vi "Teleop.vi"(10 "Match Info":T1={"Autonomous Elapsed Seconds"=0.0, "TeleOp Elapsed Seconds"=0.0, "Disabled Elapsed Seconds"=0.0, "Visited Autonomous"=FALSE, "Visited TeleOp"=FALSE, "Visited Disabled"=FALSE, "Autonomous Settings"={"Autonomous Style"=enum."Independent", "VI Refnum"=refnum}}, 11 "Call Context":T2) -> ()   [LabVIEW 2018]
doc: "This VI is called for each TeleOp packet received from the DS where the robot is not disabled. It is often used to read from the joysticks and update I/O or to update setpoints for timed control loops. It should complete and return within 20 milliseconds or it may miss DS packets."
uses:
  <vilib>/Rock Robotics/WPI/DriverStation/WPI_DriverStationDerivedRobotMode.ctl
  <vilib>/Rock Robotics/WPI/DriverStation/WPI_DriverStationMatch Info.ctl
  <vilib>/Rock Robotics/WPI/Utilities/WPI_GetSetVariantRefNum.vi
  <vilib>/Rock Robotics/Network Tables/SD Read Number.vi
panel:
  out "ENCODER VALUE LIFT 2":dbl=20.0 format="%#_13g"
  out "ENCODER VALUE Retractor":dbl=20.0 format="%#_13g"
  out "ENCODER VALUE cLIMBER":dbl=20.0 format="%#_13g"
  out "ENCODER VALUE LIFT":dbl=20.0 format="%#_13g"
  out "BR Current":dbl
  out "FL Current":dbl
  out "BL Current":dbl
  out "lim":bool
  out "Tote Offset":dbl
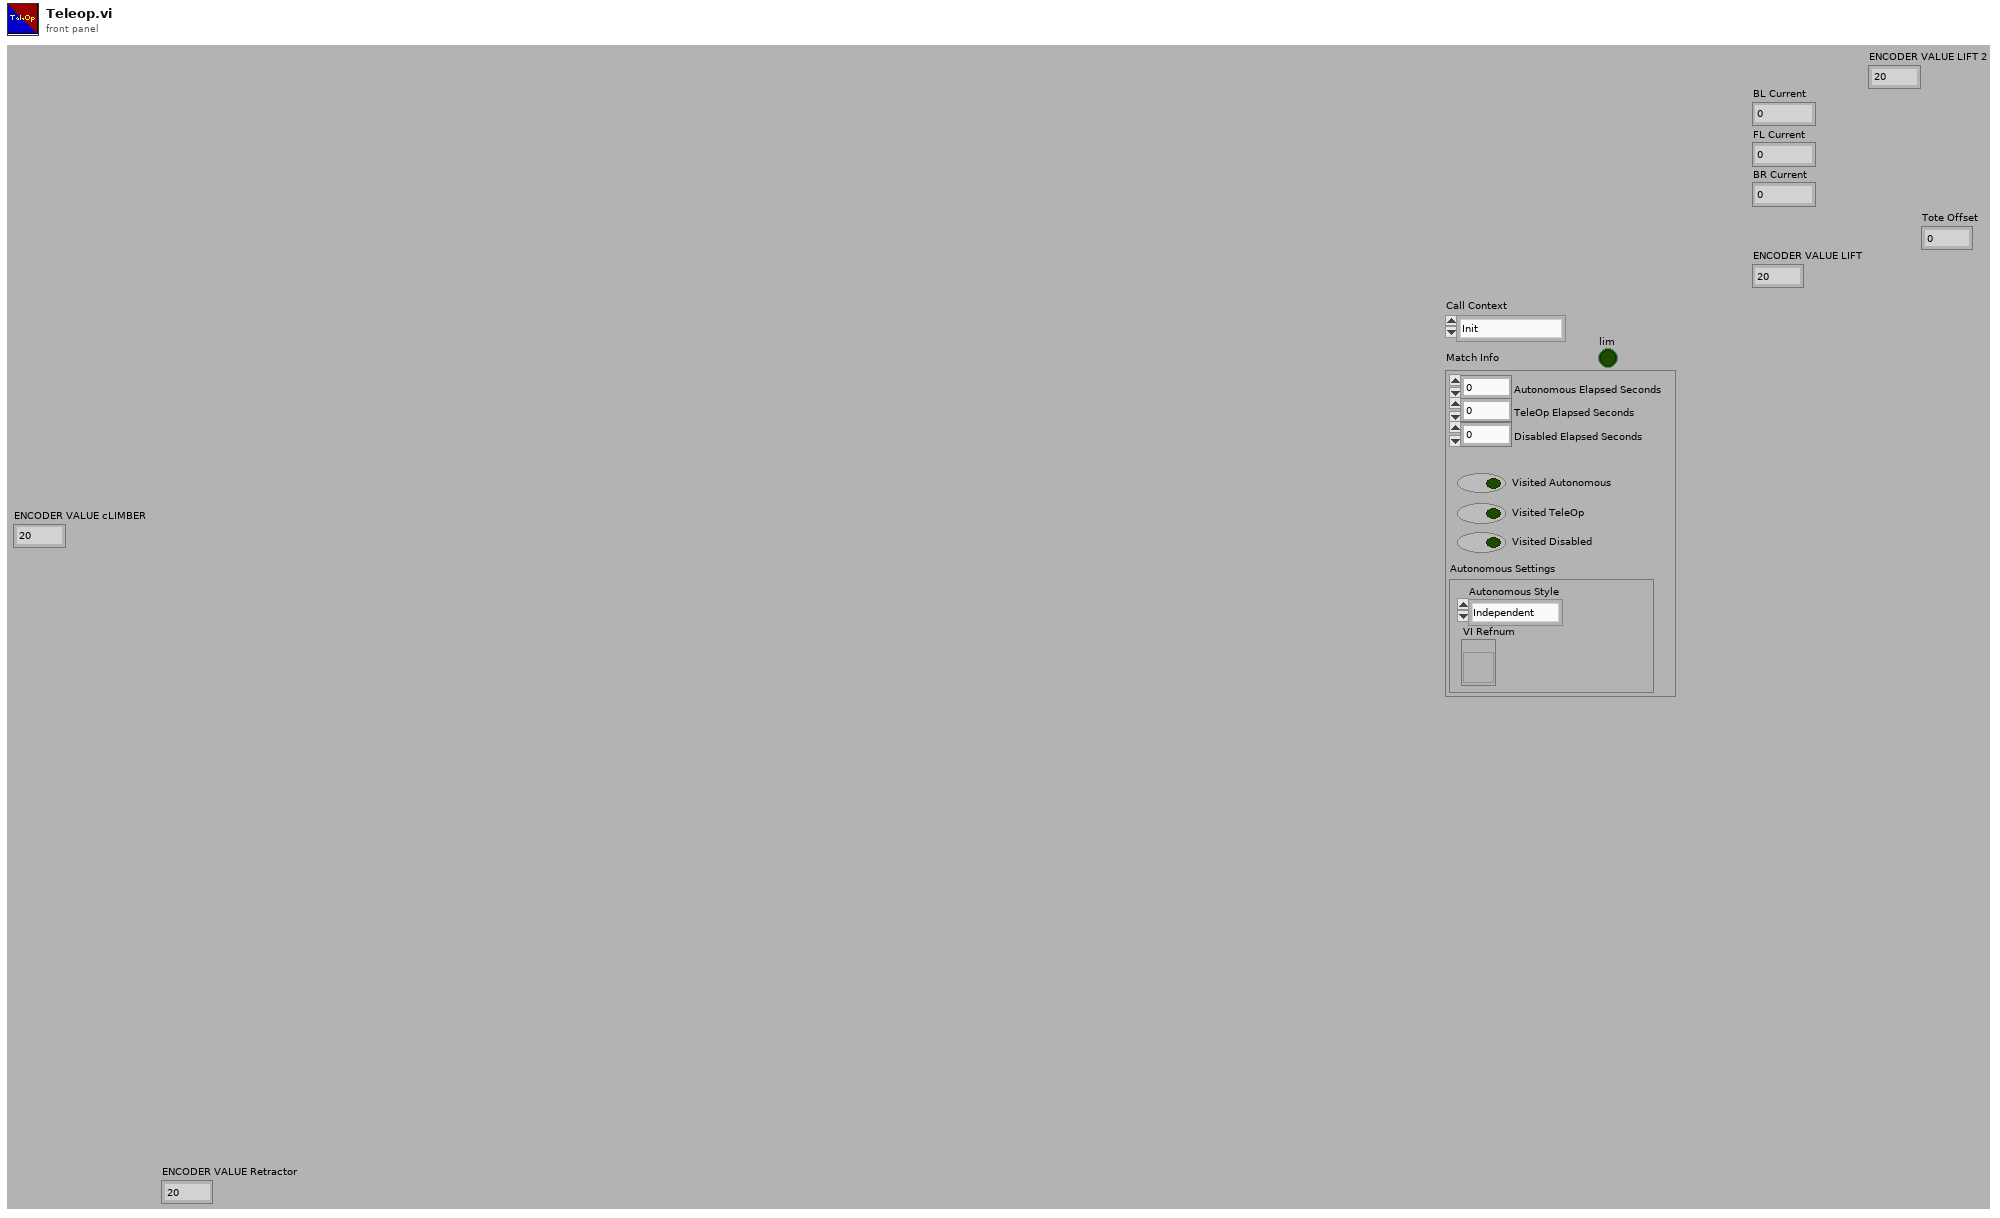
[diagram p1: front panel]
types:
  T1 = typedef "WPI_DriverStationMatch Info.ctl" = cluster{"Autonomous Elapsed Seconds":dbl, "TeleOp Elapsed Seconds":dbl, "Disabled Elapsed Seconds":dbl, "Visited Autonomous":bool, "Visited TeleOp":bool, "Visited Disabled":bool, "Autonomous Settings":cluster{"Autonomous Style":enum16{"Iterative", "Independent"}, "VI Refnum":refnum<vi>}}
  T2 = typedef "WPI_DriverStationDerivedRobotMode.ctl" = enum16{"Init", "Execute", "Stop"}
  T3 = typedef "WPI_JoystickDevRef.ctl" = cluster{"Device":T4}
  T4 = typedef "WPI_JoystickDeviceEnum.ctl" = enum16{"USB 0", "USB 1", "USB 2", "USB 3", "USB 4", "USB 5"}
  T5 = cluster{"Buttons[0]":bool, "Buttons[1]":bool, "Buttons[2]":bool, "Buttons[3]":bool, "Buttons[4]":bool, "Buttons[5]":bool, "Buttons[6]":bool, "Buttons[7]":bool, "Buttons[8]":bool, "Buttons[9]":bool, "Buttons[10]":bool, "Buttons[11]":bool}
  T6 = typedef "WPI_EncoderDevRef.ctl" = cluster{"DevStatus":errorcluster, "EncoderIndex":T7, "CounterIndex":T8, "DistancePerCount":dbl, "Decoding Type":T9}
  T7 = typedef "FPGA_EncoderIdx.ctl" = enum8{"Enc 0", "Enc 1", "Enc 2", "Enc 3", "Enc 4", "Enc 5", "Enc 6", "Enc 7", "Invalid"}
  T8 = typedef "FPGA_CounterCtrSystemIndex.ctl" = enum8{"Ctr 0", "Ctr 1", "Ctr 2", "Ctr 3", "Ctr 4", "Ctr 5", "Ctr 6", "Ctr 7", "Invalid"}
  T9 = typedef "WPI_EncoderType.ctl" = enum16{"1x", "2x", "4x"}
  T10 = cluster{"Buttons[0]":bool, "Buttons[1]":bool, "Buttons[2]":bool, "Buttons[3]":bool, "Buttons[4]":bool, "Buttons[5]":bool, "Buttons[6]":bool, "Buttons[7]":bool, "Buttons[8]":bool, "Buttons[9]":bool}
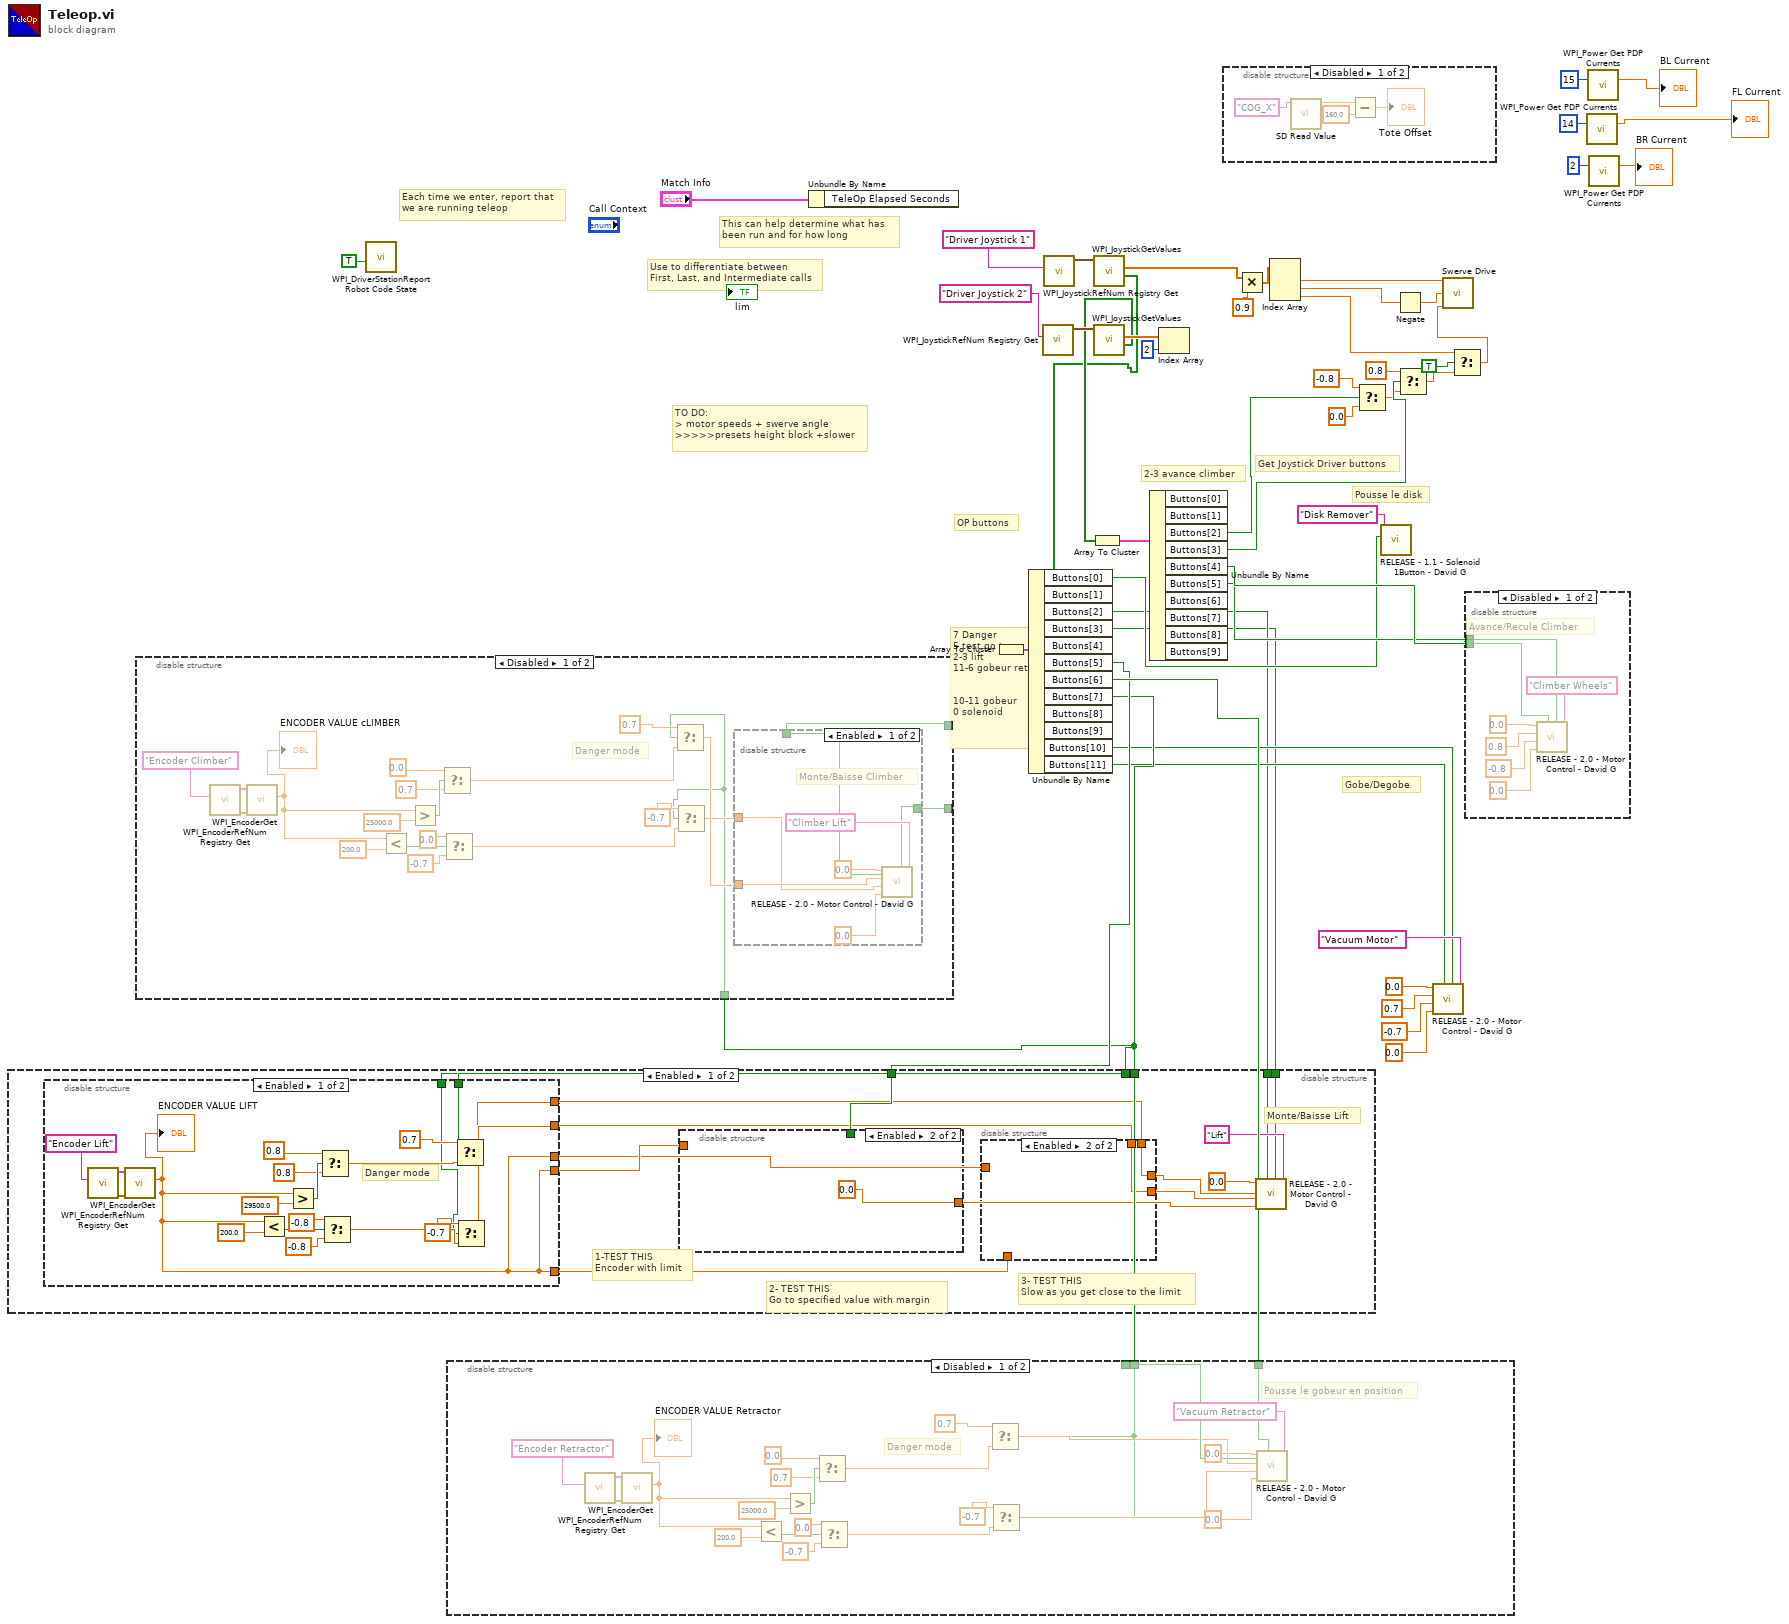
[diagram p0: block diagram]
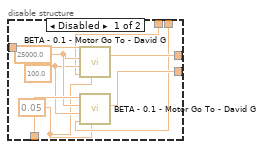
[diagram p7: hidden frame]
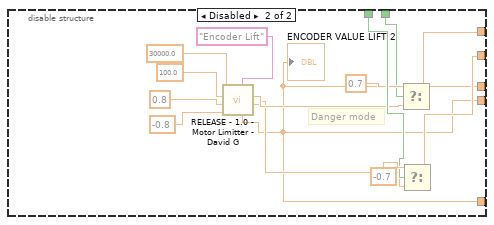
[diagram p8: hidden frame]
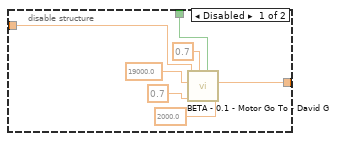
[diagram p9: hidden frame]
diagram:
  # "2-3 avance climber"
  # "7 Danger\n5 test go to\n2-3 lift\n11-6 gobeur retractor\n\n\n10-11 gobeur\n0 solenoid"
  # "OP buttons"
  # "TO DO: \n> motor speeds + swerve angle\n>>>>>presets height block +slower"
  # "Gobe/Degobe"
  # "Pousse le disk"
  # "Get Joystick Driver buttons"
  # "Each time we enter, report that\nwe are running teleop"
  # "Use to differentiate between\nFirst, Last, and Intermediate calls"
  # "This can help determine what has\nbeen run and for how long"
  n1 = call <vilib>:"WPI_DriverStationReport Robot Code State.vi"("TeleOp"=TRUE ("Autonomous")) -> ()  [unwired: 10 in, 1 out]
  n2 = Unbundle By Name("Match Info") -> ()  [unwired: 1 out]
  n3 = call <vilib>:"WPI_JoystickRefNum Registry Get.vi"("refnum name"="Driver Joystick 2") -> ("JoystickDevRef"=w46:T3)  [unwired: 1 in, 9 out]
  n4 = call <vilib>:"WPI_JoystickRefNum Registry Get.vi"("refnum name"="Driver Joystick 1") -> ("JoystickDevRef"=w48:T3)  [unwired: 1 in, 9 out]
  n5 = call <vilib>:"WPI_JoystickGetValues.vi"("JoystickDevRef"=w48) -> ("Buttons"=w6:bool[], "Axes"=w42:dbl[])  [unwired: 6 in, 3 out]
  n6 = Array To Cluster(array=w6) -> (cluster=w28:T5)
  n7 = Unbundle By Name(w28) -> ("Buttons[0]"=w3:bool, "Buttons[2]"=w2:bool, "Buttons[3]"=w1:bool, "Buttons[5]"=w22:bool, "Buttons[6]"=w23:bool, "Buttons[7]"=w21:bool, "Buttons[10]"=w4:bool, "Buttons[11]"=w5:bool)  [unwired: 4 out]
  n8 = disable-structure shown="Enabled" {
    disable-tunnel: w21 -> [w63 _]
    disable-tunnel: w21 -> [w62 _]
    disable-tunnel: w22 -> [w60 _]
    disable-tunnel: w2 -> [w52 _]
    disable-tunnel: w1 -> [w51 _]
    frame Enabled {
      # "3- TEST THIS\nSlow as you get close to the limit"
      # "1-TEST THIS\nEncoder with limit"
      # "2- TEST THIS \nGo to specified value with margin"
      # "Monte/Baisse Lift"
      n9 = disable-structure shown="Enabled" {
        disable-tunnel: [w83 w106] -> w56
        disable-tunnel: [w82 w107] -> w57
        disable-tunnel: w63 -> [w81 w99]
        disable-tunnel: w62 -> [w78 w109]
        disable-tunnel: [w77 w97] -> w61
        disable-tunnel: [w77 w97] -> w54
        disable-tunnel: [w77 w97] -> w53
        frame Enabled {
          # "Danger mode"
          n10 = call <vilib>:"WPI_EncoderRefNum Registry Get.vi"("refnum name"="Encoder Lift") -> ("error out"=w96:errorcluster, "EncoderDevRef"=w95:T6)  [unwired: 9 in]
          n11 = call <vilib>:"WPI_EncoderGet.vi"("error in (no error)"=w96, "EncoderDevRef"=w95) -> ("Distance"=w77:dbl)  [unwired: 4 in, 5 out]
          "ENCODER VALUE LIFT" <- w77
          n12 = Less?(x=w77, y=200.0 ("f")) -> (x < y?=w90:bool)
          n13 = Greater?(x=w77, y=29500.0 ("f")) -> (0:w91:bool)
          n14 = Select(t=0.8 ("f"), s=w91, f=0.8) -> (s? t:f=w85:dbl)
          n15 = Select(t=-0.8 ("f"), s=w90, f=-0.8) -> (s? t:f=w84:dbl)
          n16 = Select(t=0.7 ("f"), s=w81, f=w85) -> (s? t:f=w82:dbl)
          n17 = Select(t=-0.7 ("f"), s=w78, f=w84) -> (s? t:f=w83:dbl)
        }
        frame Disabled {
          # "Danger mode"
          n18 = call "RELEASE - 1.0 - Motor Limitter - David G.vi"("refnum name"="Encoder Lift", "Backward Speed"=-0.8 ("f"), "Forward Speed"=0.8 ("f"), "Backward Limit"=100.0 ("f"), "Forward Limit"=30000.0 ("f")) -> ("Backward Value"=w104:dbl, "Forward Value"=w105:dbl, "Encoder Value"=w97:dbl)  [unwired: 4 in]
          "ENCODER VALUE LIFT 2" <- w97
          n19 = Select(t=0.7 ("f"), s=w99, f=w105) -> (s? t:f=w107:dbl)
          n20 = Select(t=-0.7 ("f"), s=w109, f=w104) -> (s? t:f=w106:dbl)
        }
      }
      n21 = disable-structure shown="Enabled" {
        disable-tunnel: w61 -> [w114 _]
        disable-tunnel: w60 -> [w113 _]
        disable-tunnel: [w112 0.0 ("f")] -> w59
        frame Disabled {
          n22 = call "BETA - 0.1 - Motor Go To - David G.vi"("Encoder Value"=w114, "Go To"=19000.0 ("f"), "Speed"=0.7 ("f"), "Default Neutral Speed"=0.7 ("f"), "Button"=w113, "Margin (Nullable)"=2000.0 ("f")) -> ("Output Neutral Speed"=w112:dbl)  [unwired: 4 in]
        }
        frame Enabled {
        }
      }
      n23 = disable-structure shown="Enabled" {
        disable-tunnel: [w73 w76] -> w58
        disable-tunnel: w57 -> [w72 w76]
        disable-tunnel: w56 -> [w67 w75]
        disable-tunnel: [w74 w75] -> w55
        disable-tunnel: w54 -> [w71 _]
        disable-tunnel: w53 -> [w70 _]
        frame Disabled {
          w66 = 0.05 ("f")
          w68 = 100.0 ("f")
          w69 = 25000.0 ("f")
          n24 = call "BETA - 0.1 - Motor Go To - David G.vi"("Encoder Value"=w71, "Go To"=w69, "Speed"=w67, "Default Neutral Speed"=w66, "Margin (Nullable)"=w68) -> ("Output Neutral Speed"=w73:dbl)  [unwired: 5 in]
          n25 = call "BETA - 0.1 - Motor Go To - David G.vi"("Encoder Value"=w70, "Go To"=w69, "Speed"=w72, "Default Neutral Speed"=w66, "Margin (Nullable)"=w68) -> ("Output Neutral Speed"=w74:dbl)  [unwired: 5 in]
        }
        frame Enabled {
        }
      }
      n26 = call "RELEASE - 2.0 - Motor Control - David G.vi"("refnum name"="Lift", "Bouton Arrière"=w51, "Bouton Avant"=w52, "FF"=w59, "FT"=w55, "TF"=w58, "TT"=0.0 ("f")) -> ()  [unwired: 5 in]
    }
    frame Disabled {
    }
  }
  n27 = disable-structure shown="Disabled" {
    disable-tunnel: w21 -> [w121 _]
    disable-tunnel: _ -> [w120 _]
    disable-tunnel: _ -> [w119 _]
    frame Disabled {
      # "Danger mode"
      n28 = call <vilib>:"WPI_EncoderRefNum Registry Get.vi"("refnum name"="Encoder Climber") -> ("error out"=w139:errorcluster, "EncoderDevRef"=w138:T6)  [unwired: 9 in]
      n29 = call <vilib>:"WPI_EncoderGet.vi"("error in (no error)"=w139, "EncoderDevRef"=w138) -> ("Distance"=w128:dbl)  [unwired: 4 in, 5 out]
      "ENCODER VALUE cLIMBER" <- w128
      n30 = Less?(x=w128, y=200.0 ("f")) -> (x < y?=w133:bool)
      n31 = Greater?(x=w128, y=25000.0 ("f")) -> (0:w134:bool)
      n32 = Select(t=0.0 ("f"), s=w134, f=0.7) -> (s? t:f=w127:dbl)
      n33 = Select(t=0.0 ("f"), s=w133, f=-0.7) -> (s? t:f=w126:dbl)
      n34 = Select(t=0.7 ("f"), s=w121, f=w127) -> (s? t:f=w123:dbl)
      n35 = Select(t=-0.7 ("f"), s=w121, f=w126) -> (s? t:f=w122:dbl)
      n36 = disable-structure shown="Enabled" {
        disable-tunnel: w119 -> [w143 _]
        disable-tunnel: w120 -> [w142 _]
        disable-tunnel: w123 -> [w141 _]
        disable-tunnel: w122 -> [w140 _]
        frame Enabled {
          # "Monte/Baisse Climber"
          n37 = call "RELEASE - 2.0 - Motor Control - David G.vi"("refnum name"="Climber Lift", "Bouton Arrière"=w142, "Bouton Avant"=w143, "FF"=0.0 ("f"), "FT"=w140, "TF"=w141, "TT"=0.0 ("f")) -> ()  [unwired: 5 in]
        }
        frame Disabled {
        }
      }
    }
    frame Enabled {
    }
  }
  n38 = disable-structure shown="Disabled" {
    disable-tunnel: _ -> [w167 _]
    disable-tunnel: w21 -> [w148 _]
    disable-tunnel: w23 -> [w147 _]
    frame Disabled {
      # "Danger mode"
      # "Pousse le gobeur en position"
      n39 = call <vilib>:"WPI_EncoderRefNum Registry Get.vi"("refnum name"="Encoder Retractor") -> ("error out"=w166:errorcluster, "EncoderDevRef"=w165:T6)  [unwired: 9 in]
      n40 = call <vilib>:"WPI_EncoderGet.vi"("error in (no error)"=w166, "EncoderDevRef"=w165) -> ("Distance"=w155:dbl)  [unwired: 4 in, 5 out]
      "ENCODER VALUE Retractor" <- w155
      n41 = Less?(x=w155, y=200.0 ("f")) -> (x < y?=w160:bool)
      n42 = Greater?(x=w155, y=25000.0 ("f")) -> (0:w161:bool)
      n43 = Select(t=0.0 ("f"), s=w161, f=0.7) -> (s? t:f=w154:dbl)
      n44 = Select(t=0.0 ("f"), s=w160, f=-0.7) -> (s? t:f=w153:dbl)
      n45 = Select(t=0.7 ("f"), s=w148, f=w154) -> (s? t:f=w150:dbl)
      n46 = Select(t=-0.7 ("f"), s=w148, f=w153) -> (s? t:f=w149:dbl)
      n47 = call "RELEASE - 2.0 - Motor Control - David G.vi"("refnum name"="Vacuum Retractor", "Bouton Arrière"=w167, "Bouton Avant"=w147, "FF"=0.0 ("f"), "FT"=w149, "TF"=w150, "TT"=0.0 ("f")) -> ()  [unwired: 5 in]
    }
    frame Enabled {
    }
  }
  n48 = call <vilib>:"WPI_JoystickGetValues.vi"("JoystickDevRef"=w46) -> ("Buttons"=w7:bool[], "Axes"=w44:dbl[])  [unwired: 6 in, 3 out]
  n49 = Array To Cluster(array=w7) -> (cluster=w35:T10)
  n50 = Unbundle By Name(w35) -> ("Buttons[2]"=w18:bool, "Buttons[3]"=w17:bool, "Buttons[4]"=w20:bool, "Buttons[5]"=w19:bool)  [unwired: 6 out]
  n51 = Index Array(array=w44, index=2) -> ()  [unwired: 1 out]
  n52 = disable-structure shown="Disabled" {
    frame Disabled {
      n53 = call-poly <vilib>:"SD Read Value.vi"("Name"="COG_X") -> ("Numeric"=w173:dbl)  [unwired: 8 in, 2 out]
      n54 = Subtract(x=w173, y=160.0) -> (x-y=→"Tote Offset":dbl)
    }
    frame Enabled {
    }
  }
  n55 = Multiply(x=w42, y=0.9) -> (x*y=w24:dbl[])
  n56 = Index Array(array=w24) -> (element #1=w8:dbl, element #2=w26:dbl, element #3=w11:dbl)  [unwired: 3 in]
  n57 = Select(t=-0.8 ("y"), s=w18, f=0.0 ("y")) -> (s? t:f=w16:dbl)
  n58 = call "RELEASE - 1.1 - Solenoid 1Button - David G.vi"(10:w3, "refnum name"="Disk Remover") -> ()  [unwired: 10 in]
  n59 = Negate(x=w26) -> (-x=w27:dbl)
  n60 = Select(t=0.8 ("y"), s=w17, f=w16) -> (s? t:f=w12:dbl)
  n61 = call "RELEASE - 2.0 - Motor Control - David G.vi"("refnum name"="Vacuum Motor", "Bouton Arrière"=w4, "Bouton Avant"=w5, "FF"=0.0 ("f"), "FT"=-0.7 ("f"), "TF"=0.7 ("f"), "TT"=0.0 ("f")) -> ()  [unwired: 5 in]
  n62 = Select(t=w11, s=TRUE, f=w12) -> (s? t:f=w10:dbl)
  n63 = call "Swerve Drive.vi"("X"=w8, "Y"=w27, "Z"=w10) -> ()  [unwired: 13 in]
  n64 = disable-structure shown="Disabled" {
    disable-tunnel: w19 -> [w176 _]
    disable-tunnel: w20 -> [w175 _]
    frame Disabled {
      # "Avance/Recule Climber"
      n65 = call "RELEASE - 2.0 - Motor Control - David G.vi"("refnum name"="Climber Wheels", "Bouton Arrière"=w176, "Bouton Avant"=w175, "FF"=0.0 ("f"), "FT"=-0.8 ("f"), "TF"=0.8 ("f"), "TT"=0.0 ("f")) -> ()  [unwired: 5 in]
    }
    frame Enabled {
    }
  }
  n66 = call <vilib>:"WPI_Power Get PDP Currents.vi"("PDP Channel"=14) -> ("current (A)"=→"FL Current":dbl)  [unwired: 12 in, 2 out]
  n67 = call <vilib>:"WPI_Power Get PDP Currents.vi"("PDP Channel"=15) -> ("current (A)"=→"BL Current":dbl)  [unwired: 12 in, 2 out]
  n68 = call <vilib>:"WPI_Power Get PDP Currents.vi"("PDP Channel"=2) -> ("current (A)"=→"BR Current":dbl)  [unwired: 12 in, 2 out]
